vi "51 Simple Queues.vi"() -> ()   [LabVIEW 2024]
uses:
  <userlib>/1. Examples/_Subs/OpenDiagram/Open_XControl.xctl
panel:
  in  "OpenDiag":refnum<vi>(xcontrol)
  out "Value":dbl
  in  "Slide":dbl(slide) scale=0.0..10.0
  in  "Done":bool
  out "pushed?":bool
  in  "Btn":bool
  # "01 Simple Queues\nThis code shows how to use queues to make responsive front panels\n\nInstructions:\n1. Hit the Run arrow and push buttons and drag slides\n2. Watch how the program runs using the highlight execution button on the diagram"
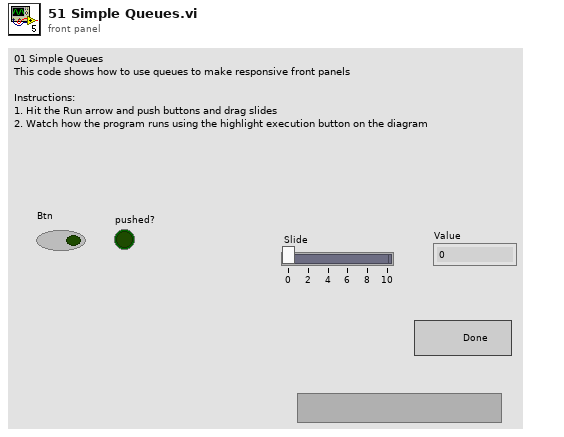
[diagram p1: front panel]
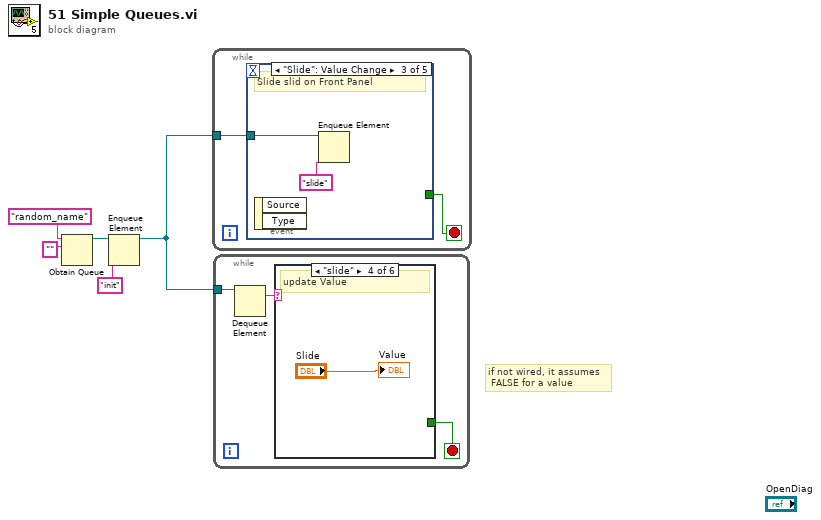
[diagram p0: block diagram]
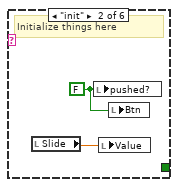
[diagram p3: hidden frame]
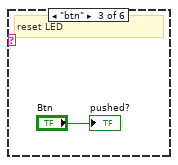
[diagram p4: hidden frame]
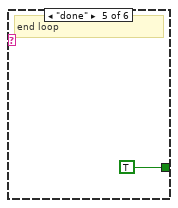
[diagram p5: hidden frame]
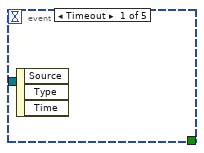
[diagram p7: hidden frame]
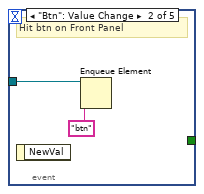
[diagram p8: hidden frame]
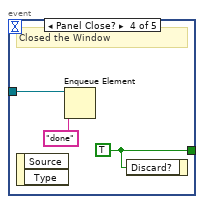
[diagram p9: hidden frame]
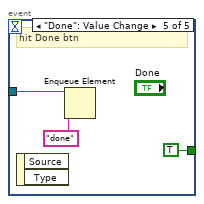
[diagram p10: hidden frame]
diagram:
  # "if not wired, it assumes\n FALSE for a value"
  n1 = Obtain Queue(name (unnamed)="random_name", element data type="") -> (queue out=w5:refnum<queue>)  [unwired: 3 in, 2 out]
  n2 = Enqueue Element(queue=w5, element="init") -> (queue out=w1:refnum<queue>)  [unwired: 2 in, 2 out]
  n3 = while {
    tunnel: w1 -> [w7]
    stop <- w6 stop-if-true
    n4 = event shown="[2] \"Slide\": Value Change" {
      selector: _ -> [_ _ _ _ _]
      dyn-events: _ -> [_ _ _ _ _]
      timeout: _ -> [_ _ _ _ _]
      tunnel: w7 -> [_ w8 w10 w13 w16]
      tunnel: [_ _ _ w12 TRUE ("Discard?")] -> w6
      event Timeout {
        n5 = event-data() -> ()  [unwired: 1 in, 3 out]
      }
      event "Btn": Value Change {
        # "Hit btn on Front Panel"
        n6 = event-data() -> ()  [unwired: 1 in, 1 out]
        n7 = Enqueue Element(queue=w8, element="btn") -> ()  [unwired: 2 in, 3 out]
      }
      event "Slide": Value Change {
        # "Slide slid on Front Panel"
        n8 = event-data() -> ()  [unwired: 1 in, 2 out]
        n9 = Enqueue Element(queue=w10, element="slide") -> ()  [unwired: 2 in, 3 out]
      }
      event Panel Close? {
        w12 = TRUE ("Discard?")
        # "Closed the Window"
        n10 = event-data() -> ()  [unwired: 1 in, 2 out]
        n11 = Enqueue Element(queue=w13, element="done") -> ()  [unwired: 2 in, 3 out]
        n12 = event-data("Discard?"=w12) -> ()  [unwired: 1 in, 1 out]
      }
      event "Done": Value Change {
        # "hit Done btn"
        n13 = event-data() -> ()  [unwired: 1 in, 2 out]
        n14 = Enqueue Element(queue=w16, element="done") -> ()  [unwired: 2 in, 3 out]
      }
    }
  }
  n15 = while {
    tunnel: w1 -> [w20]
    stop <- w18 stop-if-true
    n16 = Dequeue Element(queue=w20) -> (element=w19:string)  [unwired: 2 in, 3 out]
    n17 = case shown="\"slide\"" w19 {
      tunnel: [_ _ _ _ TRUE ("Discard?") _] -> w18
      frame Default {
      }
      frame "init" {
        w22 = FALSE ("pushed?")
        # "Initialize things here"
        n18 = local read "Slide"() -> (w21:dbl)
        n19 = local write "pushed?"(w22) -> ()
        n20 = local write "Value"(w21) -> ()
        n21 = local write "Btn"(w22) -> ()
      }
      frame "btn" {
        # "reset LED"
        "pushed?" <- "Btn"
      }
      frame "slide" {
        # "update Value"
        "Value" <- "Slide"
      }
      frame "done" {
        # "end loop"
      }
      frame "" {
      }
    }
  }
